vi "Week_4_4.1_Example_Sinewave 230V.vi"() -> ()   [LabVIEW 2015]
panel:
  in  "stop":bool
  out "Waveform Graph":dynamicdata(graph)
  in  "RMS":dbl format="%#_13g"
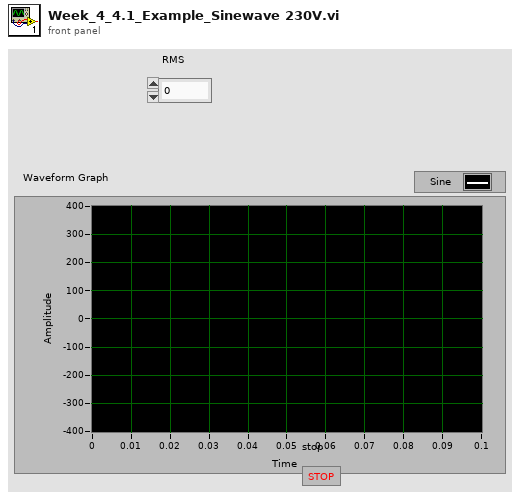
[diagram p1: front panel]
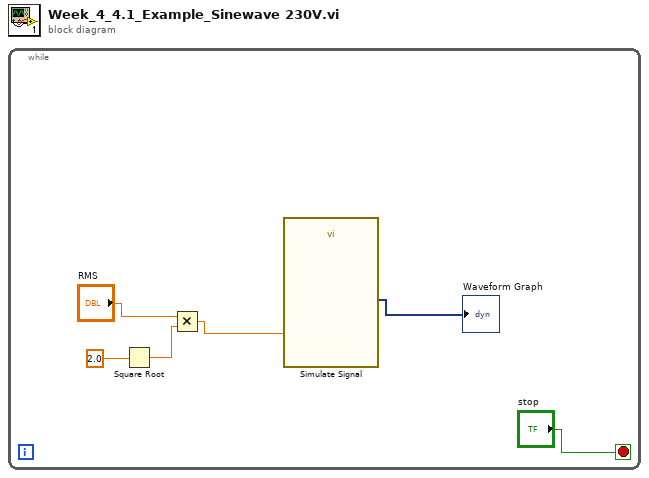
[diagram p0: block diagram]
diagram:
  n1 = while {
    stop <- "stop" stop-if-true
    n2 = Square Root(x=2.0) -> (sqrt(x)=w4:dbl)
    n3 = Multiply(x="RMS", y=w4) -> (x*y=w3:dbl)
    n4 = call "Simulate Signal"("Amplitude"=w3) -> ("Sine"=→"Waveform Graph":dynamicdata)  [unwired: 13 in, 1 out]
  }
